vi "ProdaNG.ProcessStepParams.Get.vi"(8 "error in (no error)":errorcluster, 10 "processStepId":i32, 11 "dbHandleIn":i32) -> (0 "error out":errorcluster, 2 "ProcStepParams":T1[](array[typedef]), 3 "dbHandle":i32)   [LabVIEW 2016]
doc: "This function returns a product structure for a product, which is identified by a part and a serial number.\nImportant information: The field 'individual' was taken over from the field 'allgemein' of the legacy data directly. Because of this most products have the value 0 further on and only a few the value 1. \nParameter:\nhandle is an Integer, which is returned by the function Login() at the creation of a new connection.\nwabcoPartId is the Id of the part.\nserialNumber is the serial number of the product for the part above.\nproduct is a pointer on a product structure, which is filled if the returncode is 0. The structure must be defined in the calling program.\n\nReturncodes:\n0 No error\n< 0 ORACLE Error code\n6 (ERROR_INVALID_HANDLE) in case of an invalid handle\n1403 Record does not exist"
uses:
  Controls/ProdaNG.ProcessStepParam.ctl
  Controls/ProdaNG.ProcessStepParamSize.ctl
  <vilib>/Utility/importsl/GetValueByPointer/datatype.ctl
  <vilib>/Utility/importsl/GetValueByPointer/GetValueByPointer.xnode
  prodllNG.dll
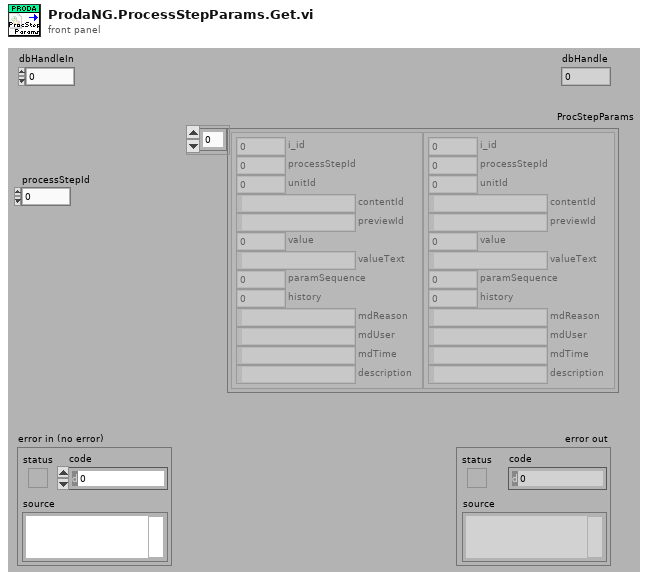
[diagram p1: front panel]
types:
  T1 = typedef "ProdaNG.ProcessStepParam.ctl" = cluster{"i_id":i32, "processStepId":i32, "unitId":i32, "contentId":string, "previewId":string, "value":dbl, "valueText":string, "paramSequence":i32, "history":i32, "mdReason":string, "mdUser":string, "mdTime":string, "description":string}
  T2 = typedef "ProdaNG.ProcessStepParamSize.ctl" = cluster{"i_id":i32, "processStepId":i32, "unitId":i32, "contentId":i32, "previewId":i32, "value":i32, "valueText":i32, "paramSequence":i32, "history":i32, "mdReason":i32, "mdUser":i32, "mdTime":i32, "description":i32}
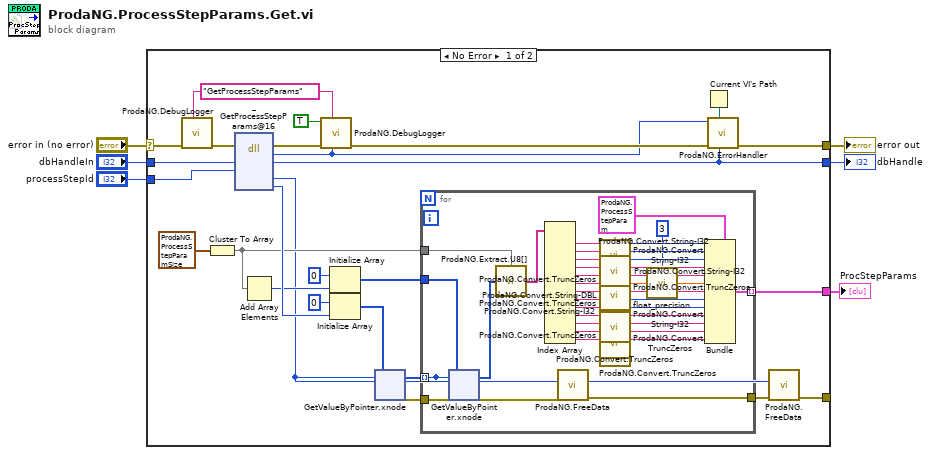
[diagram p0: block diagram]
diagram:
  n1 = case shown="No Error" "error in (no error)" {
    selector: "error in (no error)" -> [w27 w102]
    tunnel: [w32 w102] -> w5
    tunnel: "dbHandleIn" -> [w29 w101]
    tunnel: [w30 w101] -> w3
    tunnel: "processStepId" -> [w14 _]
    tunnel: [w11 _] -> w1
    tunnel: [w9 _] -> _
    frame No Error {
      w23 = "GetProcessStepParams" ("cmd")
      n2 = call "ProdaNG.DebugLogger.vi"("cmd"=w23, "error in (no error)"=w27) -> ("error out"=w26:errorcluster)  [unwired: 9 in]
      n3 = Cluster To Array(cluster=T2 {"i_id"=4, "processStepId"=4, "unitId"=4, "contentId"=16, "previewId"=16, "value"=8, "valueText"=258, "paramSequence"=4, "history"=4, "mdReason"=514, "mdUser"=22, "mdTime"=24, "description"=514} ("ProcStepSize")) -> (array=w12:i32[])
      n4 = dll-call lib="D:/svn/LineTraceSystem/SOFTWARE/sources/Database/ProdaNG/prodllNG.dll" fn="_GetProcessStepParams@16" ("ProDLL wrapper.dll:ProDLL_wrapper_GetWabcoParts_GetData")(error in=w26, "dbHandle"=w29, "processStepId"=w14) -> (error out=w25:errorcluster, "return type"=w22:i32, "dbHandle"=w30:i32, "processStepParams"=w8:u32, "countPtr"=w17:i32)  [unwired: 5 in, 1 out]
      n5 = Add Array Elements(numeric array=w12) -> (sum=w13:i32)
      n6 = call "ProdaNG.DebugLogger.vi"("return type"=w22, "cmd"=w23, "error in (no error)"=w25, "done? (F)"=TRUE) -> ("error out"=w24:errorcluster)  [unwired: 7 in]
      n7 = Initialize Array(u8 0 ("element"), w13) -> (w15:u8[])
      n8 = Initialize Array(u32 0 ("element"), w17) -> (w21:u32[])
      n9 = xnode "GetValueByPointer.xnode"("Pointer"=w8, "InputType"=w21) -> ("Output"=w18:u32[], "ErrorOut"=w19:errorcluster)  [unwired: 2 in]
      n10 = for {
        tunnel: w19 -> [w70]
        tunnel: w18 -> [w37] mode=indexing
        tunnel: w15 -> [w69]
        tunnel: w12 -> [w54]
        tunnel: [w53] -> w11 mode=indexing
        tunnel: [w36] -> w10
        n11 = xnode "GetValueByPointer.xnode"("Pointer"=w37, "InputType"=w69, "ErrorIn"=w70) -> ("Output"=w56:u8[], "ErrorOut"=w38:errorcluster)  [unwired: 1 in]
        n12 = call "ProdaNG.Extract.U8[].vi"("unsigned byte array"=w56, "Sizes"=w54) -> ("Elements"=w55:string[])
        n13 = Index Array(array=w55) -> (element #1=w58:string, element #2=w57:string, element #3=w67:string, element #4=w64:string, element #5=w62:string, element #6=w63:string, element #7=w52:string, element #8=w51:string, element #9=w48:string, element #10=w46:string, element #11=w44:string, element #12=w42:string, element #13=w39:string)  [unwired: 13 in]
        n14 = call "ProdaNG.FreeData.vi"("error in (no error)"=w38, "Pointers"=w37) -> ("error out"=w36:errorcluster)  [unwired: 9 in]
        n15 = call "ProdaNG.Convert.String-I32.vi"("unsigned byte string"=w58) -> ("32bit integer"=w60:i32)  [unwired: 10 in]
        n16 = call "ProdaNG.Convert.String-I32.vi"("unsigned byte string"=w57) -> ("32bit integer"=w59:i32)  [unwired: 10 in]
        n17 = call "ProdaNG.Convert.String-I32.vi"("unsigned byte string"=w67) -> ("32bit integer"=w66:i32)  [unwired: 10 in]
        n18 = call "ProdaNG.Convert.TruncZeros.vi"("string with \\0s"=w64) -> ("LV string"=w65:string)  [unwired: 10 in]
        n19 = call "ProdaNG.Convert.TruncZeros.vi"("string with \\0s"=w62) -> ("LV string"=w61:string)  [unwired: 10 in]
        n20 = call "ProdaNG.Convert.String-DBL.vi"("unsigned byte string"=w63) -> ("dbl integer"=w34:dbl)  [unwired: 10 in]
        n21 = call "ProdaNG.Convert.TruncZeros.vi"("string with \\0s"=w52) -> ("LV string"=w50:string)  [unwired: 10 in]
        n22 = call "ProdaNG.Convert.String-I32.vi"("unsigned byte string"=w51) -> ("32bit integer"=w49:i32)  [unwired: 10 in]
        n23 = call "ProdaNG.Convert.String-I32.vi"("unsigned byte string"=w48) -> ("32bit integer"=w47:i32)  [unwired: 10 in]
        n24 = call "ProdaNG.Convert.TruncZeros.vi"("string with \\0s"=w46) -> ("LV string"=w45:string)  [unwired: 10 in]
        n25 = call "ProdaNG.Convert.TruncZeros.vi"("string with \\0s"=w44) -> ("LV string"=w43:string)  [unwired: 10 in]
        n26 = call "ProdaNG.Convert.TruncZeros.vi"("string with \\0s"=w42) -> ("LV string"=w41:string)  [unwired: 10 in]
        n27 = call "ProdaNG.Convert.TruncZeros.vi"("string with \\0s"=w39) -> ("LV string"=w40:string)  [unwired: 10 in]
        n28 = call "float_precision.vi"("input"=w34, "precision"=3) -> ("output"=w33:dbl)
        n29 = Bundle(cluster=T1 {"i_id"=0, "processStepId"=0, "unitId"=0, "contentId"="", "previewId"="", "value"=0.0, "valueText"="", "paramSequence"=0, "history"=0, "mdReason"="", "mdUser"="", "mdTime"="", "description"=""} ("ProcessStepParam"), "i_id"=w60, "processStepId"=w59, "unitId"=w66, "contentId"=w65, "previewId"=w61, "value"=w33, "valueText"=w50, "paramSequence"=w49, "history"=w47, "mdReason"=w45, "mdUser"=w43, "mdTime"=w41, "description"=w40) -> (w53:T1)
      }
      n30 = Current VI's Path() -> (path=w31:path)
      n31 = call "ProdaNG.ErrorHandler.vi"("dbHandleIn"=w30, "Path"=w31, "error in"=w24, "output_parameter"=w22) -> ("error out"=w32:errorcluster)  [unwired: 7 in]
      n32 = call "ProdaNG.FreeData.vi"("error in (no error)"=w10, "Pointers"=w8) -> ("error out"=w9:errorcluster)  [unwired: 9 in]
    }
    frame Error {
    }
  }
  "error out" <- w5
  "dbHandle" <- w3
  "ProcStepParams" <- w1
